vi "BIO_do_connect_accept.vi"(8 "error in (no error)":errorcluster, 9 "Timeout (10000ms)":u32=10000, 11 "BIO in":refnum<class "BIO.lvclass">) -> (0 "error out":errorcluster, 3 "BIO out":refnum<class "BIO.lvclass">)   [LabVIEW 2013, in "OpenSSL Socket.lvlib" / "BIO.lvclass"]
uses:
  BIO.lvclass
  SSL-Lib/SSL-Lib.lvclass
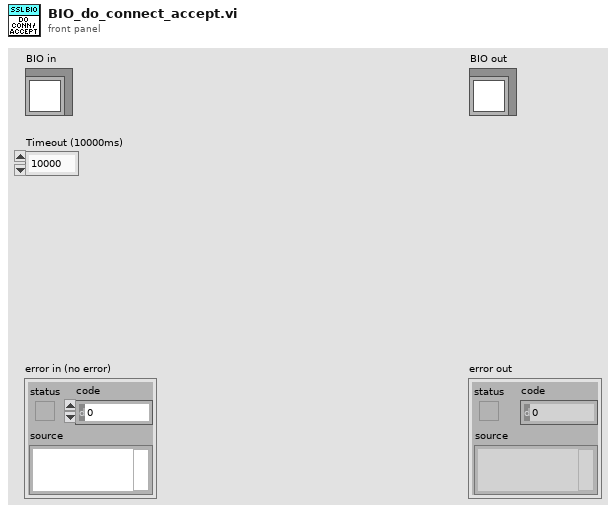
[diagram p1: front panel]
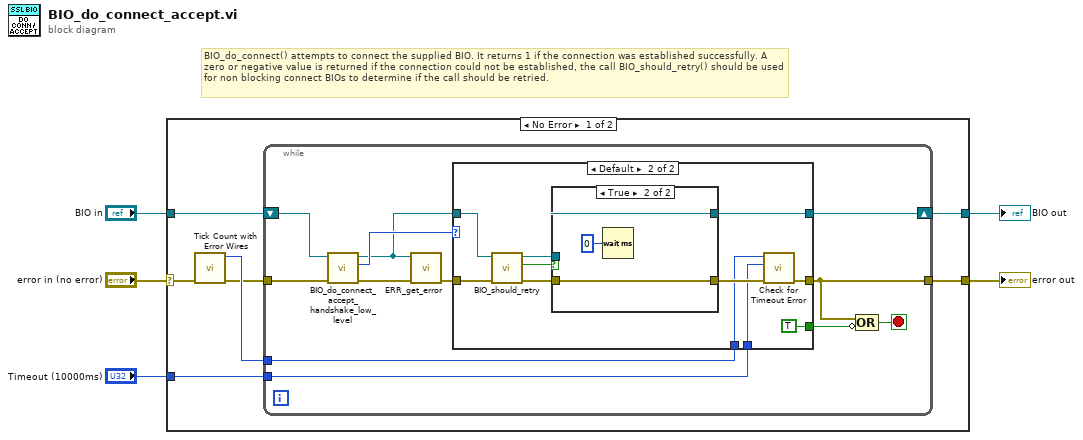
[diagram p0: block diagram]
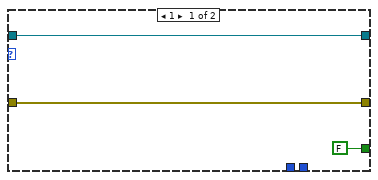
[diagram p2: hidden frame]
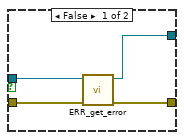
[diagram p3: hidden frame]
diagram:
  # "BIO_do_connect() attempts to connect the supplied BIO. It returns 1 if the connection was established successfully. A zero or negative value is returned if the connection could not be established, the call BIO_should_retry() should be used for non blocking connect BIOs to determine if the call should be retried."
  n1 = case shown="No Error" "error in (no error)" {
    selector: "error in (no error)" -> [w11 w47]
    tunnel: [w12 w47] -> w4
    tunnel: [w7 w46] -> w2
    tunnel: "BIO in" -> [w8 w46]
    tunnel: "Timeout (10000ms)" -> [w9 _]
    frame No Error {
      n2 = call "Tick Count with Error Wires.vi"("error in (no error)"=w11) -> ("error out"=w6:errorcluster, "millisecond timer value"=w10:u32)  [unwired: 9 in]
      n3 = while {
        tunnel: w10 -> [w21]
        tunnel: w9 -> [w22]
        tunnel: [w20] -> w12
        tunnel: w6 -> [w17]
        shift-right: [w19] -> w7
        shift-left: w8 -> [w18]
        stop <- w24 stop-if-true
        n4 = call "BIO_do_connect_accept_handshake_low_level.vi"("error in (no error)"=w17, "BIO in"=w18) -> ("error out"=w15:errorcluster, "return type"=w16:i32, "BIO out"=w14:refnum<class "BIO.lvclass">)  [unwired: 7 in]
        n5 = call "ERR_get_error.vi"("error in (no error)"=w15, "SSL-Lib in"=w14) -> ("error out"=w13:errorcluster)  [unwired: 8 in, 1 out]
        n6 = case shown="Default" w16 {
          tunnel: w13 -> [w27 w38]
          tunnel: w14 -> [w26 w32]
          tunnel: [w26 w35] -> w19
          tunnel: [w27 w30] -> w20
          tunnel: [FALSE ("Should retry") TRUE ("Should retry")] -> w23
          tunnel: w22 -> [_ w29]
          tunnel: w21 -> [_ w28]
          frame 1 {
          }
          frame Default {
            n7 = call "BIO_should_retry.vi"("error in (no error)"=w38, "BIO in"=w32) -> ("error out"=w37:errorcluster, "Should retry"=w33:bool, "BIO out"=w36:refnum<class "BIO.lvclass">)  [unwired: 7 in]
            n8 = case shown="True" w33 {
              tunnel: w37 -> [w42 w44]
              tunnel: w36 -> [w41 w45]
              tunnel: [w40 w45] -> w35
              tunnel: [w39 w44] -> w31
              frame False {
                n9 = call "ERR_get_error.vi"("error in (no error)"=w42, "SSL-Lib in"=w41) -> ("error out"=w39:errorcluster, "SSL-Lib out"=w40:refnum<class "BIO.lvclass">)  [unwired: 8 in]
              }
              frame True {
                n10 = Wait (ms)(milliseconds to wait=u32 0) -> ()  [unwired: 1 out]
              }
            }
            n11 = call "Check for Timeout Error.vi"("error in (no error)"=w31, "Timeout (10000ms)"=w29, "t0"=w28) -> ("error out"=w30:errorcluster)  [unwired: 8 in]
          }
        }
        n12 = Compound Arithmetic op=OR(w20, invert w23) -> (w24:bool)
      }
    }
    frame Error {
    }
  }
  "error out" <- w4
  "BIO out" <- w2
